vi "target_main_mem.vi"() -> ()   [LabVIEW 2023]
uses:
  <vilib>/rvi/Emulation/niFpgaGetClockAttributes.vi
  <vilib>/rvi/Emulation/niFpgaSctlEmulationGetInTimedLoop.vi
  <vilib>/rvi/Emulation/niFpgaEmulationReportErrorSimple.vi
  <vilib>/rvi/Emulation/niFpgaProcessEmulError.vi
  <vilib>/eio/utilities/niEioResolveVilibRelativePath.vi
  <vilib>/rvi/interface/RandomDataEmulation/niFpgaRandomDataHandleErrors.vi
  <vilib>/rvi/Memory/Memory_Emulation/nirvimemoryEmulation.vi
  <vilib>/rvi/Memory/Memory_Emulation/nirvimemoryFastEmulation.vi
  <vilib>/rvi/DataTransferAndStorage/Container/Common/niFpgaContainerGetUniqueNameForEmu.vi
  <vilib>/rvi/Memory/Memory_Emulation/niFpgaMemoryEmulationCacheClearOnFirstRun.vi
  <vilib>/rvi/Memory/Memory_Emulation/nirvimemoryEmulationManagerCache_MakeExclusive.vi
  <vilib>/rvi/Memory/Memory_Emulation/niFpgaMemoryEmulationValidateCache.vi
  <vilib>/rvi/Memory/Memory_Emulation/nirvimemoryEmulationManagerCache_InsertValue.vi
  <vilib>/Utility/error.llb/Clear Errors.vi
  <vilib>/rvi/Memory/Memory_Emulation/nirvimemoryEmulationManagerCache_ReleaseExclusive.vi
  <vilib>/rvi/Memory/Memory_Emulation/nirvimemoryEmulationManagerCache_GetValue.vi
  <vilib>/rvi/Emulation/niFpgaEmulationIsFPGAContextNoSignature.vi
  <vilib>/rvi/Memory/Memory_Emulation/nirvimemoryEmulationManagerCache_SetValue.vi
  <vilib>/rvi/Emulation/niFpgaSctlEmulationResourceMgr.vi
  <vilib>/rvi/errors/nirviReportUnexpectedCaseInternalError (U32).vi
  <vilib>/rvi/Emulation/niFpgaCriticalErrorInLSC.vi
  <vilib>/rvi/DataTransferAndStorage/Container/XNode/niFpgaContainer.xnode
  <vilib>/rvi/interface/RandomDataEmulation/nirviRandomDataFpgaReadWriteTemplate.vi
panel:
  in  "att7":fxp<+/-,20,5>
  in  "att6":fxp<+/-,20,5>
  in  "att5":fxp<+/-,20,5>
  in  "att4":fxp<+/-,20,5>
  in  "att3":fxp<+/-,20,5>
  in  "att2":fxp<+/-,20,5>
  in  "att1":fxp<+/-,20,5>
  in  "Vps1":fxp<+/-,20,5> format="%.3f"
  in  "Vps2":fxp<+/-,20,5> format="%.3f"
  in  "Vps3":fxp<+/-,20,5> format="%.3f"
  in  "Vps4":fxp<+/-,20,5> format="%.3f"
  in  "Vps5":fxp<+/-,20,5> format="%.3f"
  in  "Vps6":fxp<+/-,20,5> format="%.3f"
  in  "Direct Set Analogue 1":bool
  in  "Direct Set Analogue 2":bool
  out "Tick Ref":u32
  in  "Set Analogue 2":bool
  in  "Set Analogue 1":bool
  in  "Set Analogue 0":bool
  in  "FPGA Status Update Loop Time (uSec)":u32=100
  out "att 1":fxp<+/-,20,5> format="%.2g"
  out "att 2":fxp<+/-,20,5> format="%.2g"
  out "att 3":fxp<+/-,20,5> format="%.2g"
  out "att 4":fxp<+/-,20,5> format="%.2g"
  out "att 5":fxp<+/-,20,5> format="%.2g"
  out "att 6":fxp<+/-,20,5> format="%.2g"
  out "att 7":fxp<+/-,20,5> format="%.2g"
  out "Vps 1":fxp<+/-,23,10> format="%.2g"
  out "Vps 2":fxp<+/-,23,10> format="%.2g"
  out "Vps 3":fxp<+/-,23,10> format="%.2g"
  out "Vps 4":fxp<+/-,23,10> format="%.2g"
  out "Vps 5":fxp<+/-,23,10> format="%.2g"
  out "Vps 6":fxp<+/-,23,10> format="%.2g"
  in  "Load Actions Digitals":bool
  in  "Load Actions Analogue 2":bool
  in  "Load Actions Analogue 1":bool
  out "pin 6":fxp<+/-,20,5> format="%.2g"
  out "pin 5":fxp<+/-,20,5> format="%.2g"
  out "pin 4":fxp<+/-,20,5> format="%.2g"
  out "pin 3":fxp<+/-,20,5> format="%.2g"
  out "pin 2":fxp<+/-,20,5> format="%.2g"
  out "pin 1":fxp<+/-,20,5> format="%.2g"
  in  "Flush FIFO":bool
  out "Addr Analogue 1":u32
  out "Addr Analogue 2":u32
  out "Addr Digitals":u32
  out "Addr Analogue 0":u32
  in  "Abort":bool
  in  "Status Code":u8
  out "Num of Actions Digitals":u32
  out "Num of Actions Analogue 2":u32
  out "Num of Actions Analogue 1":u32
  out "Num of Actions Analogue 0":u32
  in  "Trigger Experiment":bool
  in  "Analogue 2":u32
  in  "Analogue 1":u32
  in  "Analogue 0":u32
  in  "Digitals":u32
  out "FPGA Target Clock Tick":u32
  in  "FPGA Tick Reset":bool
  in  "Load Actions Analogue 0":bool
  # "Line States"
  # "Laser Toggle Status"
  # "Command from Host"
  # "Action States"
  # "A0: Optical Switch Pins"
  # "A1: Phase Shifter Voltages"
  # "A2: Attenuator Pins"
  # "Direct Set A1"
  # "Direct Set A2"
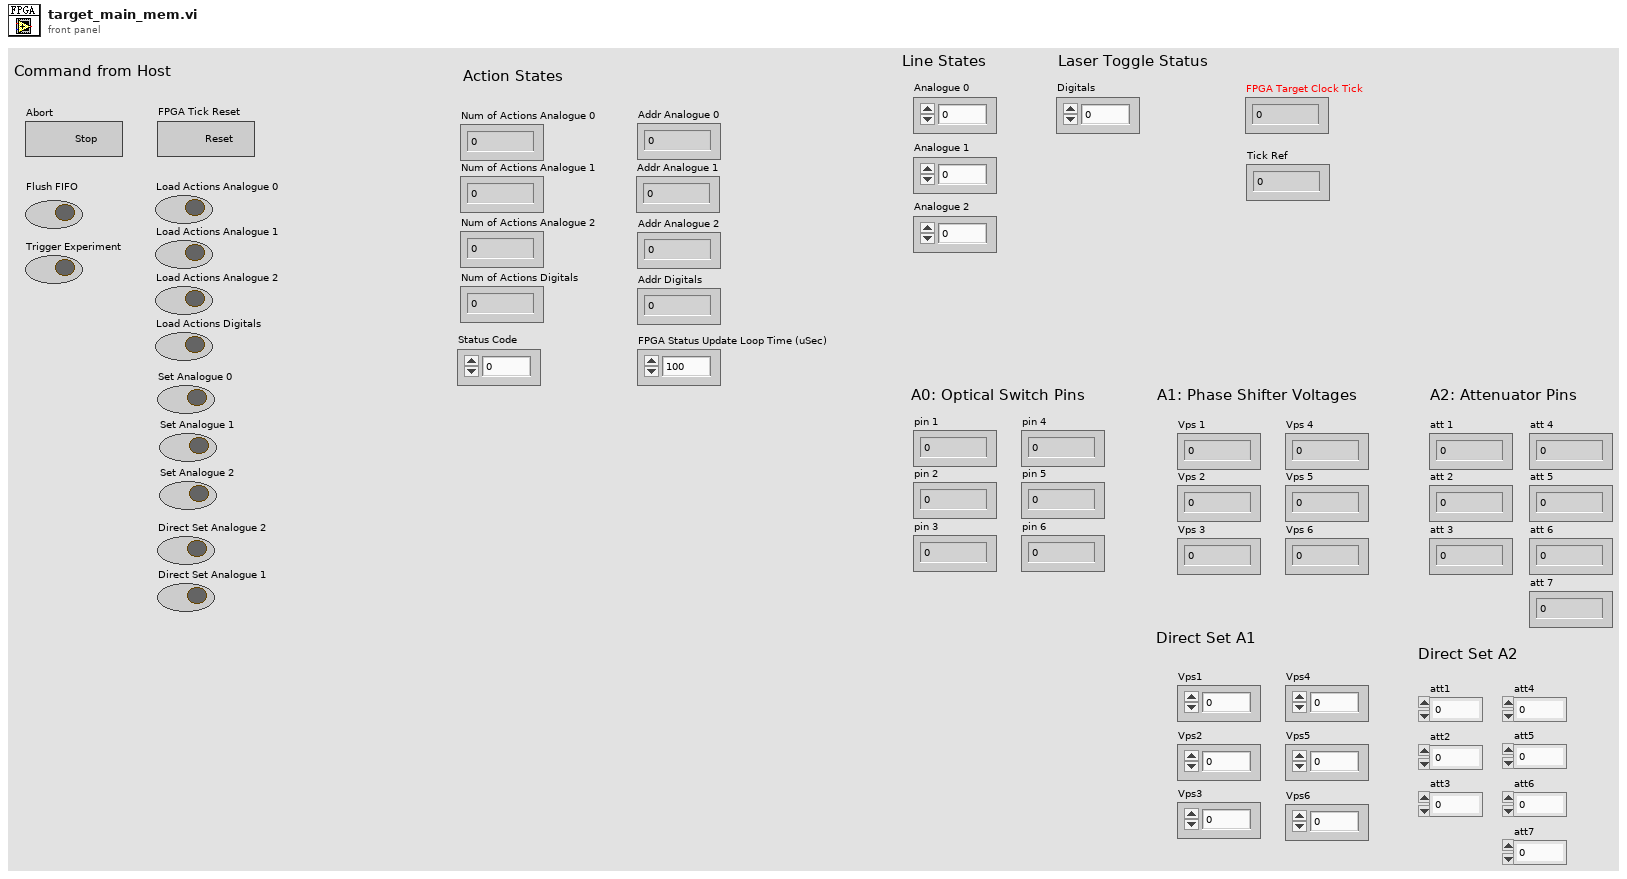
[diagram p1: front panel]
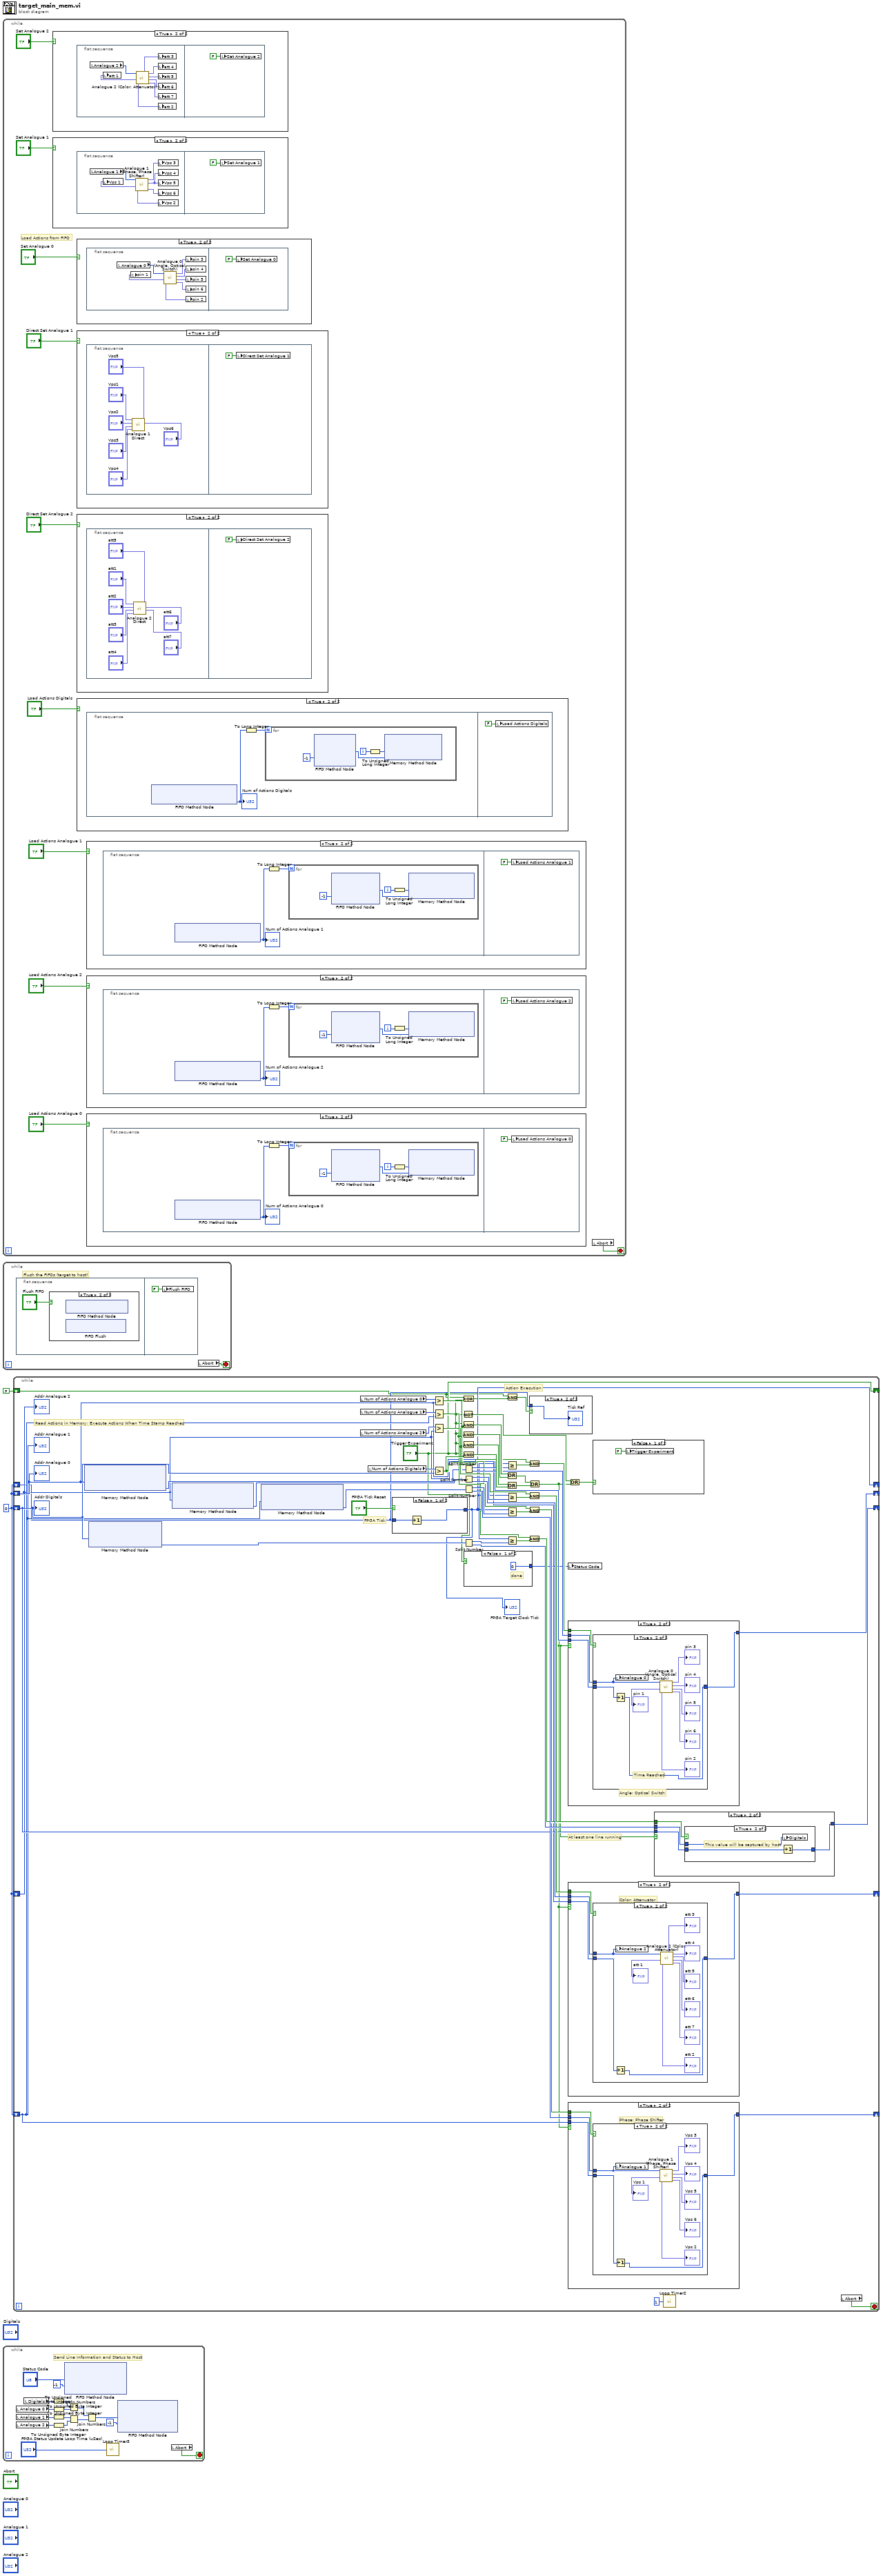
[diagram p0: block diagram]
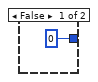
[diagram p3: hidden frame]
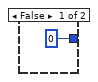
[diagram p5: hidden frame]
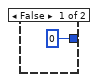
[diagram p7: hidden frame]
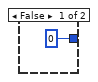
[diagram p9: hidden frame]
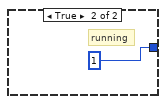
[diagram p12: hidden frame]
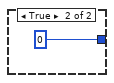
[diagram p13: hidden frame]
diagram:
  w2 = u32 0
  n1 = while {
    stop <- w12 stop-if-true
    # "Load Actions from FIFO"
    n2 = case shown="True" "Set Analogue 2" {
      frame False {
      }
      frame True {
        n3 = flat-sequence {
          frame #0 {
            n4 = local read "Analogue 2"() -> (w35:u32)
            n5 = call "Analogue 2 (Color, Attenuator).vi"("Laser Color"=w35) -> ("att 7"=w28:fxp<+/-,20,5>, "att 6"=w29:fxp<+/-,20,5>, "att 5"=w30:fxp<+/-,20,5>, "att 4"=w31:fxp<+/-,20,5>, "att 3"=w32:fxp<+/-,20,5>, "att 2"=w33:fxp<+/-,20,5>, "att 1"=w34:fxp<+/-,20,5>)  [unwired: 4 in]
            n6 = local write "att 1"(w34) -> ()
            n7 = local write "att 3"(w32) -> ()
            n8 = local write "att 4"(w31) -> ()
            n9 = local write "att 5"(w30) -> ()
            n10 = local write "att 6"(w29) -> ()
            n11 = local write "att 7"(w28) -> ()
            n12 = local write "att 2"(w33) -> ()
          }
          frame #1 {
            n13 = local write "Set Analogue 2"(FALSE ("Set Analogue 2")) -> ()
          }
        }
      }
    }
    n14 = case shown="True" "Set Analogue 1" {
      frame False {
      }
      frame True {
        n15 = flat-sequence {
          frame #0 {
            n16 = local read "Analogue 1"() -> (w42:u32)
            n17 = call "Analogue 1 (Phase, Phase Shifter).vi"("Phase Shifter"=w42) -> ("Vps 6"=w37:fxp<+/-,23,10>, "Vps 4"=w38:fxp<+/-,23,10>, "Vps 3"=w39:fxp<+/-,23,10>, "Vps 2"=w40:fxp<+/-,23,10>, "Vps 1"=w41:fxp<+/-,23,10>)  [unwired: 5 in, 1 out]
            n18 = local write "Vps 1"(w41) -> ()
            n19 = local write "Vps 3"(w39) -> ()
            n20 = local write "Vps 4"(w38) -> ()
            n21 = local write "Vps 5"(w38) -> ()
            n22 = local write "Vps 6"(w37) -> ()
            n23 = local write "Vps 2"(w40) -> ()
          }
          frame #1 {
            n24 = local write "Set Analogue 1"(FALSE ("Set Analogue 1")) -> ()
          }
        }
      }
    }
    n25 = case shown="True" "Set Analogue 0" {
      frame False {
      }
      frame True {
        n26 = flat-sequence {
          frame #0 {
            n27 = local read "Analogue 0"() -> (w50:u32)
            n28 = call "Analogue 0 (Angle, Optical Switch).vi"("Port Number"=w50) -> ("pin 6"=w44:fxp<+/-,20,5>, "pin 5"=w45:fxp<+/-,20,5>, "pin 4"=w46:fxp<+/-,20,5>, "pin 3"=w47:fxp<+/-,20,5>, "pin 2"=w48:fxp<+/-,20,5>, "pin 1"=w49:fxp<+/-,20,5>)  [unwired: 5 in]
            n29 = local write "pin 1"(w49) -> ()
            n30 = local write "pin 3"(w47) -> ()
            n31 = local write "pin 4"(w46) -> ()
            n32 = local write "pin 5"(w45) -> ()
            n33 = local write "pin 6"(w44) -> ()
            n34 = local write "pin 2"(w48) -> ()
          }
          frame #1 {
            n35 = local write "Set Analogue 0"(FALSE ("Set Analogue 0")) -> ()
          }
        }
      }
    }
    n36 = case shown="True" "Direct Set Analogue 1" {
      frame False {
      }
      frame True {
        n37 = flat-sequence {
          frame #0 {
            n38 = call "Analogue 1 Direct.vi"("Vps 6"="Vps6", "Vps 5"="Vps5", "Vps 4"="Vps4", "Vps 3"="Vps3", "Vps 2"="Vps2", "Vps 1"="Vps1") -> ()  [unwired: 6 in]
          }
          frame #1 {
            n39 = local write "Direct Set Analogue 1"(FALSE ("Direct Set Analogue 1")) -> ()
          }
        }
      }
    }
    n40 = case shown="True" "Direct Set Analogue 2" {
      frame False {
      }
      frame True {
        n41 = flat-sequence {
          frame #0 {
            n42 = call "Analogue 2 Direct.vi"("att 7"="att7", "att 6"="att6", "att 5"="att5", "att 4"="att4", "att 3"="att3", "att 2"="att2", "att 1"="att1") -> ()  [unwired: 5 in]
          }
          frame #1 {
            n43 = local write "Direct Set Analogue 2"(FALSE ("Direct Set Analogue 2")) -> ()
          }
        }
      }
    }
    n44 = case shown="True" "Load Actions Digitals" {
      frame False {
      }
      frame True {
        n45 = flat-sequence {
          frame #0 {
            n46 = xnode ("FIFO Method Node")() -> ("Number of Elements to Read"=w53:u32)  [unwired: 1 in, 1 out]
            "Num of Actions Digitals" <- w53
            n47 = To Long Integer(number=w53) -> (32bit integer=w52:i32)
            n48 = for {
              N: w52 -> [_]
              i -> [w57]
              n49 = xnode ("FIFO Method Node")("Timeout"=-1) -> ("Element"=w55:u64)  [unwired: 1 in, 2 out]
              n50 = To Unsigned Long Integer(number=w57) -> (unsigned 32bit integer=w56:u32)
              n51 = xnode ("Memory Method Node")("Address"=w56, "Data"=w55) -> ()  [unwired: 1 in, 1 out]
            }
          }
          frame #1 {
            n52 = local write "Load Actions Digitals"(FALSE ("Load Actions Digital 0")) -> ()
          }
        }
      }
    }
    n53 = case shown="True" "Load Actions Analogue 1" {
      frame False {
      }
      frame True {
        n54 = flat-sequence {
          frame #0 {
            n55 = xnode ("FIFO Method Node")() -> ("Number of Elements to Read"=w67:u32)  [unwired: 1 in, 1 out]
            "Num of Actions Analogue 1" <- w67
            n56 = To Long Integer(number=w67) -> (32bit integer=w66:i32)
            n57 = for {
              N: w66 -> [_]
              i -> [w71]
              n58 = xnode ("FIFO Method Node")("Timeout"=-1) -> ("Element"=w68:u64)  [unwired: 1 in, 2 out]
              n59 = To Unsigned Long Integer(number=w71) -> (unsigned 32bit integer=w70:u32)
              n60 = xnode ("Memory Method Node")("Address"=w70, "Data"=w68) -> ()  [unwired: 1 in, 1 out]
            }
          }
          frame #1 {
            n61 = local write "Load Actions Analogue 1"(FALSE ("Load Actions Analogue 1")) -> ()
          }
        }
      }
    }
    n62 = case shown="True" "Load Actions Analogue 2" {
      frame False {
      }
      frame True {
        n63 = flat-sequence {
          frame #0 {
            n64 = xnode ("FIFO Method Node")() -> ("Number of Elements to Read"=w60:u32)  [unwired: 1 in, 1 out]
            "Num of Actions Analogue 2" <- w60
            n65 = To Long Integer(number=w60) -> (32bit integer=w59:i32)
            n66 = for {
              N: w59 -> [_]
              i -> [w64]
              n67 = xnode ("FIFO Method Node")("Timeout"=-1) -> ("Element"=w62:u64)  [unwired: 1 in, 2 out]
              n68 = To Unsigned Long Integer(number=w64) -> (unsigned 32bit integer=w63:u32)
              n69 = xnode ("Memory Method Node")("Address"=w63, "Data"=w62) -> ()  [unwired: 1 in, 1 out]
            }
          }
          frame #1 {
            n70 = local write "Load Actions Analogue 2"(FALSE ("Load Actions Analogue 2")) -> ()
          }
        }
      }
    }
    n71 = case shown="True" "Load Actions Analogue 0" {
      frame False {
      }
      frame True {
        n72 = flat-sequence {
          frame #0 {
            n73 = xnode ("FIFO Method Node")() -> ("Number of Elements to Read"=w73:u32)  [unwired: 1 in, 1 out]
            "Num of Actions Analogue 0" <- w73
            n74 = To Long Integer(number=w73) -> (32bit integer=w74:i32)
            n75 = for {
              N: w74 -> [_]
              i -> [w78]
              n76 = xnode ("FIFO Method Node")("Timeout"=-1) -> ("Element"=w75:u64)  [unwired: 1 in, 2 out]
              n77 = To Unsigned Long Integer(number=w78) -> (unsigned 32bit integer=w77:u32)
              n78 = xnode ("Memory Method Node")("Address"=w77, "Data"=w75) -> ()  [unwired: 1 in, 1 out]
            }
          }
          frame #1 {
            n79 = local write "Load Actions Analogue 0"(FALSE) -> ()
          }
        }
      }
    }
    n80 = local read "Abort"() -> (w12:bool)
  }
  n81 = while {
    stop <- w80 stop-if-true
    # "Flush the FIFOs (target to host)"
    n82 = flat-sequence {
      frame #0 {
        n83 = case shown="True" "Flush FIFO" {
          frame False {
          }
          frame True {
            n84 = xnode ("FIFO Method Node")() -> ()  [unwired: 1 in, 1 out]
            n85 = xnode ("FIFO Flush")() -> ()  [unwired: 1 in, 1 out]
          }
        }
      }
      frame #1 {
        n86 = local write "Flush FIFO"(FALSE ("Flush FIFO")) -> ()
      }
    }
    n87 = local read "Abort"() -> (w80:bool)
  }
  n88 = while {
    stop <- w85 stop-if-true
    # "Send Line Information and Status to Host"
    n89 = local read "Analogue 0"() -> (w97:u32)
    n90 = local read "Analogue 1"() -> (w96:u32)
    n91 = local read "Analogue 2"() -> (w95:u32)
    n92 = local read "Digitals"() -> (w84:u32)
    n93 = To Unsigned Byte Integer(number=w84) -> (unsigned 8bit integer=w94:u8)
    n94 = To Unsigned Byte Integer(number=w97) -> (unsigned 8bit integer=w93:u8)
    n95 = To Unsigned Byte Integer(number=w96) -> (unsigned 8bit integer=w92:u8)
    n96 = To Unsigned Byte Integer(number=w95) -> (unsigned 8bit integer=w91:u8)
    n97 = xnode ("FIFO Method Node")("Element"="Status Code", "Timeout"=-1) -> ()  [unwired: 1 in, 2 out]
    n98 = Join Numbers(hi=w94, lo=w93) -> ((hi.lo)=w89:u16)
    n99 = Join Numbers(hi=w92, lo=w91) -> ((hi.lo)=w90:u16)
    n100 = Join Numbers(hi=w89, lo=w90) -> ((hi.lo)=w88:u32)
    n101 = call "Loop Timer3"("Count(uSec)"="FPGA Status Update Loop Time (uSec)") -> ()  [unwired: 1 out]
    n102 = xnode ("FIFO Method Node")("Element"=w88, "Timeout"=-1) -> ()  [unwired: 1 in, 2 out]
    n103 = local read "Abort"() -> (w85:bool)
  }
  n104 = while {
    shift-right: [w105] -> _
    shift-left: w2 -> [w102]
    shift-right: [w122] -> _
    shift-left: w2 -> [w118]
    shift-right: [w121] -> _
    shift-left: w2 -> [w117]
    shift-right: [w120] -> _
    shift-left: w2 -> [w106]
    shift-right: [w119] -> _
    shift-left: w2 -> [w116]
    shift-right: ["Trigger Experiment"] -> _
    shift-left: FALSE ("Trigger Experiment") -> [w100]
    stop <- w108 stop-if-true
    # "FPGA Tick"
    # "Read Actions in Memory; Execute Actions When Time Stamp Reaches"
    # "At least one line running"
    # "Action Execution"
    n105 = xnode ("Memory Method Node")("Address"=w118) -> ("Data"=w113:u64)  [unwired: 1 in, 1 out]
    n106 = xnode ("Memory Method Node")("Address"=w117) -> ("Data"=w112:u64)  [unwired: 1 in, 1 out]
    n107 = xnode ("Memory Method Node")("Address"=w106) -> ("Data"=w111:u64)  [unwired: 1 in, 1 out]
    n108 = xnode ("Memory Method Node")("Address"=w116) -> ("Data"=w110:u64)  [unwired: 1 in, 1 out]
    n109 = local read "Num of Actions Analogue 0"() -> (w148:u32)
    n110 = local read "Num of Actions Analogue 1"() -> (w147:u32)
    n111 = local read "Num of Actions Analogue 2"() -> (w146:u32)
    n112 = local read "Num of Actions Digitals"() -> (w145:u32)
    n113 = case shown="False" "FPGA Tick Reset" {
      tunnel: [w214 u32 0] -> w105
      tunnel: w102 -> [w213 _]
      frame False {
        n114 = Increment(x=w213) -> (x+1=w214:u32)
      }
      frame True {
      }
    }
    "FPGA Target Clock Tick" <- w105
    n115 = Greater?(x=w148, y=w118) -> (0:w128:bool)
    n116 = Greater?(x=w147, y=w116) -> (0:w127:bool)
    n117 = Greater?(x=w146, y=w106) -> (0:w124:bool)
    n118 = Greater?(x=w145, y=w117) -> (0:w133:bool)
    n119 = Not(x="Trigger Experiment") -> (.not. x?=w107:bool)
    n120 = Exclusive Or(1:"Trigger Experiment", 2:w100) -> (0:w101:bool)
    n121 = And(x="Trigger Experiment", y=w128) -> (x .and. y?=w153:bool)
    n122 = And(x="Trigger Experiment", y=w127) -> (x .and. y?=w152:bool)
    n123 = And(x="Trigger Experiment", y=w124) -> (x .and. y?=w151:bool)
    n124 = And(x="Trigger Experiment", y=w133) -> (x .and. y?=w150:bool)
    n125 = Split Number(x=w113) -> (hi(x)=w142:u32, lo(x)=w141:u32)
    n126 = Split Number(x=w111) -> (hi(x)=w135:u32, lo(x)=w134:u32)
    n127 = Split Number(x=w110) -> (hi(x)=w137:u32, lo(x)=w136:u32)
    n128 = Split Number(x=w112) -> (hi(x)=w140:u32, lo(x)=w139:u32)
    n129 = case shown="False" "Trigger Experiment" {
      tunnel: [u8 0 ("Status Code") u8 1 ("Status Code")] -> w115
      frame False {
        # "done"
      }
      frame True {
        # "running"
      }
    }
    n130 = Or(x=w153, y=w152) -> (x .or. y?=w144:bool)
    n131 = Or(x=w151, y=w150) -> (x .or. y?=w143:bool)
    n132 = Greater Or Equal?(x=w105, y=w142) -> (x >= y?=w131:bool)
    n133 = Greater Or Equal?(x=w105, y=w135) -> (x >= y?=w125:bool)
    n134 = Greater Or Equal?(x=w105, y=w137) -> (x >= y?=w129:bool)
    n135 = Greater Or Equal?(x=w105, y=w140) -> (x >= y?=w138:bool)
    n136 = And(x=w100, y=w101) -> (x .and. y?=w99:bool)
    n137 = And(x=w128, y=w131) -> (x .and. y?=w130:bool)
    n138 = And(x=w124, y=w125) -> (x .and. y?=w123:bool)
    n139 = And(x=w127, y=w129) -> (x .and. y?=w126:bool)
    n140 = And(x=w133, y=w138) -> (x .and. y?=w132:bool)
    n141 = Or(x=w144, y=w143) -> (x .or. y?=w104:bool)
    n142 = case shown="True" w99 {
      tunnel: w102 -> [_ w154]
      frame False {
      }
      frame True {
        "Tick Ref" <- w154
      }
    }
    n143 = local write "Status Code"(w115) -> ()
    n144 = case shown="True" w104 {
      tunnel: w130 -> [_ w199]
      tunnel: w141 -> [_ w198]
      tunnel: w118 -> [_ w197]
      tunnel: [u32 0 ("Addr Analogue 0") w196] -> w122
      frame False {
      }
      frame True {
        # "Angle: Optical Switch"
        n145 = case shown="True" w199 {
          tunnel: w198 -> [_ w207]
          tunnel: [w200 w209] -> w196
          tunnel: w197 -> [w200 w208]
          frame False {
            # "Time Not Reached or Actions Done"
          }
          frame True {
            # "Time Reached"
            n146 = Increment(x=w208) -> (x+1=w209:u32)
            n147 = local write "Analogue 0"(w207) -> ()
            n148 = call "Analogue 0 (Angle, Optical Switch).vi"("Port Number"=w207) -> ("pin 6"=→"pin 6":fxp<+/-,20,5>, "pin 5"=→"pin 5":fxp<+/-,20,5>, "pin 4"=→"pin 4":fxp<+/-,20,5>, "pin 3"=→"pin 3":fxp<+/-,20,5>, "pin 2"=→"pin 2":fxp<+/-,20,5>, "pin 1"=→"pin 1":fxp<+/-,20,5>)  [unwired: 5 in]
          }
        }
      }
    }
    n149 = case shown="True" w104 {
      tunnel: w106 -> [_ w159]
      tunnel: w123 -> [_ w158]
      tunnel: w134 -> [_ w157]
      tunnel: [u32 0 ("Addr Analogue 2") w156] -> w120
      frame False {
      }
      frame True {
        # "Color: Attenuator"
        n150 = case shown="True" w158 {
          tunnel: w157 -> [_ w161]
          tunnel: [w160 w170] -> w156
          tunnel: w159 -> [w160 w169]
          frame False {
          }
          frame True {
            n151 = Increment(x=w169) -> (x+1=w170:u32)
            n152 = local write "Analogue 2"(w161) -> ()
            n153 = call "Analogue 2 (Color, Attenuator).vi"("Laser Color"=w161) -> ("att 7"=→"att 7":fxp<+/-,20,5>, "att 6"=→"att 6":fxp<+/-,20,5>, "att 5"=→"att 5":fxp<+/-,20,5>, "att 4"=→"att 4":fxp<+/-,20,5>, "att 3"=→"att 3":fxp<+/-,20,5>, "att 2"=→"att 2":fxp<+/-,20,5>, "att 1"=→"att 1":fxp<+/-,20,5>)  [unwired: 4 in]
          }
        }
      }
    }
    n154 = case shown="True" w104 {
      tunnel: w116 -> [_ w175]
      tunnel: w126 -> [_ w174]
      tunnel: w136 -> [_ w173]
      tunnel: [u32 0 ("Addr Analogue 1") w172] -> w119
      frame False {
      }
      frame True {
        # "Phase: Phase Shifter"
        n155 = case shown="True" w174 {
          tunnel: w173 -> [_ w177]
          tunnel: [w176 w185] -> w172
          tunnel: w175 -> [w176 w184]
          frame False {
          }
          frame True {
            n156 = Increment(x=w184) -> (x+1=w185:u32)
            n157 = local write "Analogue 1"(w177) -> ()
            n158 = call "Analogue 1 (Phase, Phase Shifter).vi"("Phase Shifter"=w177) -> ("Vps 6"=→"Vps 6":fxp<+/-,23,10>, "Vps 5"=→"Vps 5":fxp<+/-,23,10>, "Vps 4"=→"Vps 4":fxp<+/-,23,10>, "Vps 3"=→"Vps 3":fxp<+/-,23,10>, "Vps 2"=→"Vps 2":fxp<+/-,23,10>, "Vps 1"=→"Vps 1":fxp<+/-,23,10>)  [unwired: 5 in]
          }
        }
      }
    }
    n159 = Or(x=w107, y=w104) -> (x .or. y?=w114:bool)
    n160 = case shown="False" w114 {
      frame False {
        n161 = local write "Trigger Experiment"(FALSE ("Trigger Experiment")) -> ()
      }
      frame True {
      }
    }
    n162 = case shown="True" w104 {
      tunnel: w117 -> [_ w190]
      tunnel: w132 -> [_ w189]
      tunnel: w139 -> [_ w188]
      tunnel: [u32 0 ("Addr Digital 0") w187] -> w121
      frame False {
      }
      frame True {
        n163 = case shown="True" w189 {
          tunnel: w188 -> [_ w194]
          tunnel: [w191 w193] -> w187
          tunnel: w190 -> [w191 w192]
          frame False {
          }
          frame True {
            # "This value will be captured by host"
            n164 = Increment(x=w192) -> (x+1=w193:u32)
            n165 = local write "Digitals"(w194) -> ()
          }
        }
      }
    }
    n166 = call "Loop Timer2"("Count(uSec)"=u32 1) -> ()  [unwired: 1 out]
    n167 = local read "Abort"() -> (w108:bool)
    "Addr Analogue 0" <- w118
    "Addr Digitals" <- w117
    "Addr Analogue 2" <- w106
    "Addr Analogue 1" <- w116
  }
